vi "Test Configuration File Isolate by Context.vi"(8 "error in (no error)":errorcluster, 11 "Configuration File Process Interface Test In":refnum<class "Configuration File Process Interface Test.lvclass">) -> (0 "error out":errorcluster, 3 "Configuration File Process Interface Test Out":refnum<class "Configuration File Process Interface Test.lvclass">)   [LabVIEW 2020, in "Configuration File Process Interface Test.lvclass"]
uses:
  Configuration File Process Interface Test.lvclass
  Framework/Application/Application.lvclass
  Mock Configurable Process/Mock Configurable Process.lvclass
  <vilib>/Asteme/LUnit/Test Case.lvclass
  C:/Users/anton/Documents/GitHub/Triarc-Framework/source/Framework/Process/Process.lvclass
  C:/Users/anton/Documents/GitHub/Triarc-Framework/source/Framework/Base/Base.lvclass
  C:/Users/anton/Documents/GitHub/Triarc-Framework/source/Framework/Configuration File/Configuration File.lvclass
  C:/Users/anton/Documents/GitHub/Triarc-Framework/source/Framework/Configuration/Configuration.lvclass
  C:/Users/anton/Documents/GitHub/Triarc-Framework/source/Framework/Error Handler Interface/Error Handler Interface.lvclass
  C:/Users/anton/Documents/GitHub/Triarc-Framework/source/Framework/Logging/Logging.lvclass
  C:/Users/anton/Documents/GitHub/Triarc-Framework/source/Framework Test/Mock Configurable Process/Mock Configurable Process.lvclass
  C:/Users/anton/Documents/GitHub/Triarc-Framework/source/Framework Test/Configuration Interface Test/Configuration Interface Test.lvclass
  C:/Program Files (x86)/National Instruments/LabVIEW 2020/vi.lib/Asteme/LUnit/Test Case.lvclass
  C:/Users/anton/Documents/GitHub/Triarc-Framework/source/Framework Test/Configuration File Process Interface Test/Configuration File Process Interface Test.lvclass
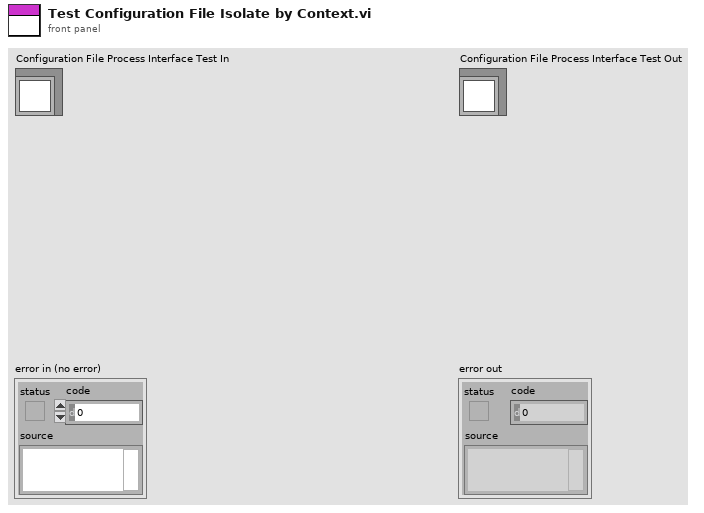
[diagram p1: front panel]
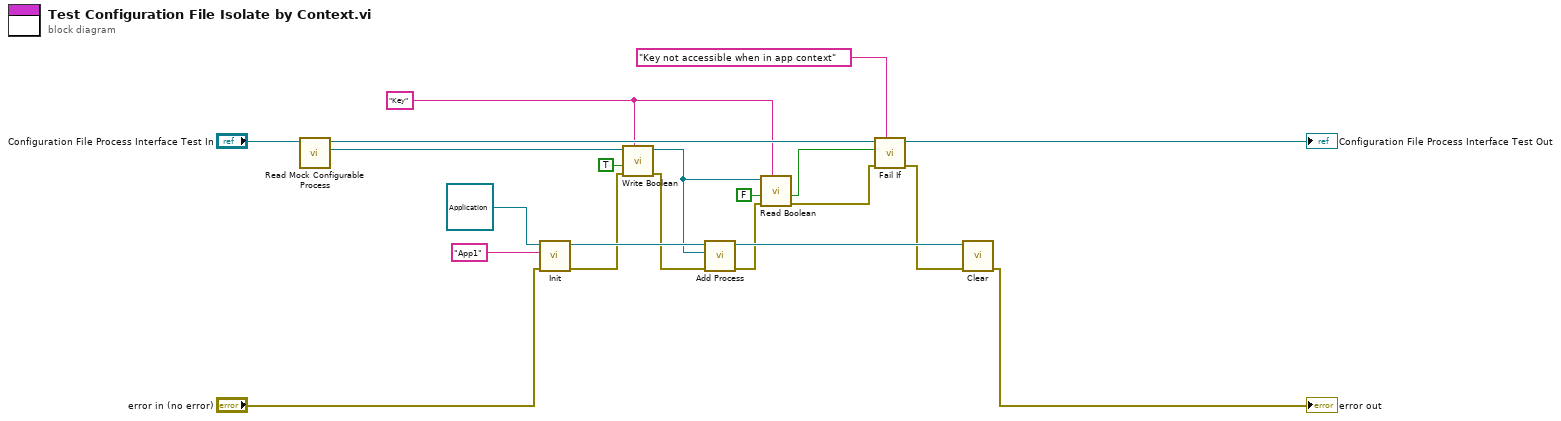
[diagram p0: block diagram]
diagram:
  w6 = "Key" ("key")
  n1 = call "Read Mock Configurable Process.vi"("Configuration File Process Interface Test in"="Configuration File Process Interface Test In") -> ("Mock Configurable.lvclass"=w16:refnum<class "Mock Configurable Process.lvclass">, "Configuration File Process Interface Test out"=w11:refnum<class "Configuration File Process Interface Test.lvclass">)  [unwired: 9 in]
  n2 = call-dynamic "Init.vi"("error in (no error)"="error in (no error)", "Name"="App1", "Process In"=refnum<class "Application.lvclass"> refnum ("Application.lvclass")) -> ("error out"=w8:errorcluster, "Process Out"=w18:refnum<class "Application.lvclass">)  [unwired: 7 in]
  n3 = call-dynamic "Write Boolean.vi"("key"=w6, "error in (no error)"=w8, "Value"=TRUE, "Configuration File In"=w16) -> ("error out"=w7:errorcluster, "Configuration File Out"=w9:refnum<class "Mock Configurable Process.lvclass">)  [unwired: 6 in]
  n4 = call "Add Process.vi"("error in (no error)"=w7, "Process"=w9, "Rig In"=w18) -> ("error out"=w14:errorcluster, "Rig Out"=w20:refnum<class "Application.lvclass">)  [unwired: 7 in]
  n5 = call-dynamic "Read Boolean.vi"("key"=w6, "error in (no error)"=w14, "default value"=FALSE ("Value"), "Configuration File In"=w9) -> ("error out"=w13:errorcluster, "value"=w4:bool)  [unwired: 5 in, 1 out]
  n6 = call <vilib>:"Fail If.vi"("Description"="Key not accessible when in app context", "error in (no error)"=w13, "Fail?"=w4, "Test Case In"=w11) -> ("error out"=w12:errorcluster, "Test Case Out"=→"Configuration File Process Interface Test Out":refnum<class "Configuration File Process Interface Test.lvclass">)  [unwired: 6 in]
  n7 = call-dynamic "Clear.vi"("error in (no error)"=w12, "Application In"=w20) -> ("error out"=→"error out":errorcluster)  [unwired: 9 in]
